vi "Remove Sibling.vi"(8 "error in (no error)":errorcluster, 10 "Sibling":refnum<data-value>, 11 "NodeRef In":refnum<data-value>) -> (0 "error out":errorcluster, 3 "NodeRef":refnum<data-value>)   [LabVIEW 2020, in "PicoG-ParserLexer.lvlib" / "Node.lvclass"]
doc: "Removes the <b>Sibling</b> by getting the current <b>NodeRef</b>'s parent and calling Remove Child on the parent.\n\n<b>Error Codes:</b>\n<b>1556</b>: The node reference is invalid; nodes must be initialized with Ctor\n<b>15</b>: The <b>Sibling</b> node was not found as a sibling of this node."
uses:
  Node.lvclass
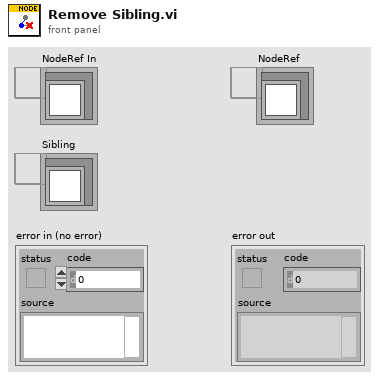
[diagram p1: front panel]
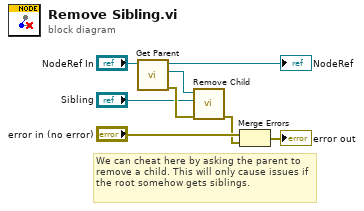
[diagram p0: block diagram]
diagram:
  # "We can cheat here by asking the parent to remove a child. This will only cause issues if the root somehow gets siblings."
  n1 = call "Get Parent.vi"("NodeRef In"="NodeRef In") -> ("error out"=w8:errorcluster, "Parent"=w5:refnum<data-value>, "NodeRef"=→"NodeRef":refnum<data-value>)  [unwired: 8 in]
  n2 = call "Remove Child.vi"("error in (no error)"=w8, "Child"="Sibling", "NodeRef In"=w5) -> ("error out"=w1:errorcluster)  [unwired: 7 in, 1 out]
  n3 = Merge Errors("error in (no error)", w1) -> (→"error out":errorcluster)
